vi "Force Anode Puge--SubVI.vi"(7 "Anode Request Events":T1, 8 "error in (no error)":errorcluster, 9 "Purge Settings in":T4, 10 "Purge State in":T3, 11 "Refnum in":refnum<k21>) -> (0 "error out":errorcluster, 1 "Purge Settings out":T4, 2 "Purge State out 2":T3, 3 "Refnum out":refnum<k21>)   [LabVIEW 2024, in "Anode.lvlib"]
uses:
  Anode.lvlib
  Purge Strategy--cluster.ctl
  Purge Strategy--enum.ctl
  Purge Valve State--cluster.ctl
  Request Events--cluster.ctl
  Stop Argument--cluster.ctl
  Show Panel Argument--cluster.ctl
  Hide Panel Argument--cluster.ctl
  Get Module Execution Status Argument--cluster.ctl
  Show Diagram Argument--cluster.ctl
  Change Panel Argument--cluster.ctl
  <vilib>/MGI/Panel Manager/Panel/Panel/Panel.lvclass
  Set Anode Inlet Pressure SP Argument--cluster.ctl
  Initialise Pressure Regulator Interface Argument--cluster.ctl
  Modbus Config--cluster.ctl
  Start Polling Pressure Regulator Status Argument--cluster.ctl
  Stop Polling Pressure Regulator Status Argument--cluster.ctl
  Read Pressure Regulator Status Argument--cluster.ctl
  Set Pressure Regulator Control Function Argument--cluster.ctl
  Modbus Flexi-Flow API/Control Function Values--enum.ctl
  Set Anode Inlet Flow SP Argument--cluster.ctl
  Set Anode Inlet Valve State Argument--cluster.ctl
  Anode Solenoid Valve--enum.ctl
  Wake Connection Helper Loop Argument--cluster.ctl
  Set Anode Gas Supply Valve Argument--cluster.ctl
  Set Purge Valve Argument--cluster.ctl
  Set Purge Strategy Argument--cluster.ctl
  Wake Purge Strategy Helper Loop Argument--cluster.ctl
  Update Purge Strategy Settings Argument--cluster.ctl
  Wake Purge Helper Loop Argument--cluster.ctl
  Wake Recirculation Pump Helper Loop Argument--cluster.ctl
  Sleep Recirculation Pump Helper Loop Argument--cluster.ctl
  Set Pump Speed SP Argument--cluster.ctl
  Set Pump Enable State Argument--cluster.ctl
  Set Pump Speed Control Mode Argument--cluster.ctl
  Update Purge Strategy Helper Loop Argument--cluster.ctl
  Force Purge Argument--cluster.ctl
  Reset Counter Argument--cluster.ctl
  Wake H2 Sensor Loop Argument--cluster.ctl
  Sleep H2 Sensor Loop Argument--cluster.ctl
  Start H2 Sensor Measurement Argument--cluster.ctl
  Stop H2 Sensor Measurement Argument--cluster.ctl
  <vilib>/DAQmx/write.llb/DAQmx Write (Digital Bool 1Line 1Point).vi
  <vilib>/DAQmx/miscellaneous.llb/DAQmx Fill In Error Info.vi
  Modbus Flexi-Flow API/Bronkhorst Flexi-Flow ModbusTCP API.lvlib
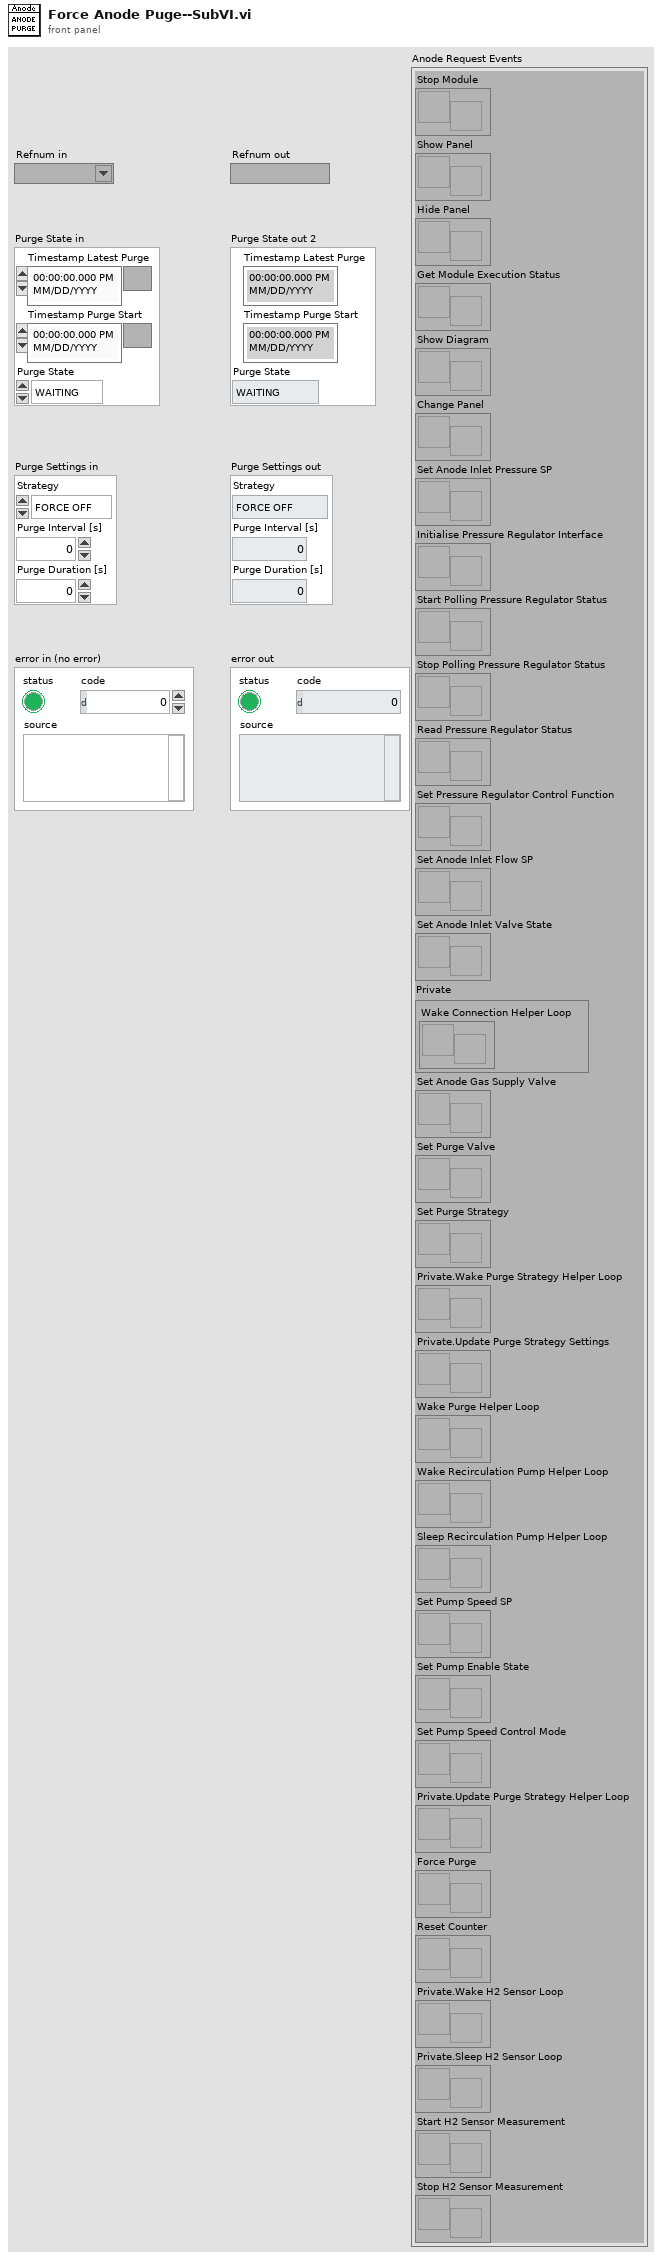
[diagram p1: front panel]
types:
  T1 = typedef "Anode.lvlib/Request Events--cluster.ctl" = cluster{"Stop Module":refnum<user-event>, "Show Panel":refnum<user-event>, "Hide Panel":refnum<user-event>, "Get Module Execution Status":refnum<user-event>, "Show Diagram":refnum<user-event>, "Change Panel":refnum<user-event>, "Set Anode Inlet Pressure SP":refnum<user-event>, "Initialise Pressure Regulator Interface":refnum<user-event>, "Start Polling Pressure Regulator Status":refnum<user-event>, "Stop Polling Pressure Regulator Status":refnum<user-event>, "Read Pressure Regulator Status":refnum<user-event>, "Set Pressure Regulator Control Function":refnum<user-event>, "Set Anode Inlet Flow SP":refnum<user-event>, "Set Anode Inlet Valve State":refnum<user-event>, "Private":cluster{"Wake Connection Helper Loop":refnum<user-event>}, "Set Anode Gas Supply Valve":refnum<user-event>, "Set Purge Valve":refnum<user-event>, "Set Purge Strategy":refnum<user-event>, "Private.Wake Purge Strategy Helper Loop":refnum<user-event>, "Private.Update Purge Strategy Settings":refnum<user-event>, "Wake Purge Helper Loop":refnum<user-event>, "Wake Recirculation Pump Helper Loop":refnum<user-event>, "Sleep Recirculation Pump Helper Loop":refnum<user-event>, "Set Pump Speed SP":refnum<user-event>, "Set Pump Enable State":refnum<user-event>, "Set Pump Speed Control Mode":refnum<user-event>, "Private.Update Purge Strategy Helper Loop":refnum<user-event>, "Force Purge":refnum<user-event>, "Reset Counter":refnum<user-event>, "Private.Wake H2 Sensor Loop":refnum<user-event>, "Private.Sleep H2 Sensor Loop":refnum<user-event>, "Start H2 Sensor Measurement":refnum<user-event>, "Stop H2 Sensor Measurement":refnum<user-event>}
  T2 = typedef "Anode.lvlib/Purge Valve State--cluster.ctl" = enum16{"WAITING", "PURGING"}
  T3 = cluster{"Timestamp Latest Purge":timestamp, "Timestamp Purge Start":timestamp, "Purge State":T2}
  T4 = typedef "Anode.lvlib/Purge Strategy--cluster.ctl" = cluster{"Strategy":T5, "Purge Interval [s]":dbl, "Purge Duration [s]":dbl}
  T5 = typedef "Anode.lvlib/Purge Strategy--enum.ctl" = enum16{"FORCE OFF", "FORCE ON", "TIMED"}
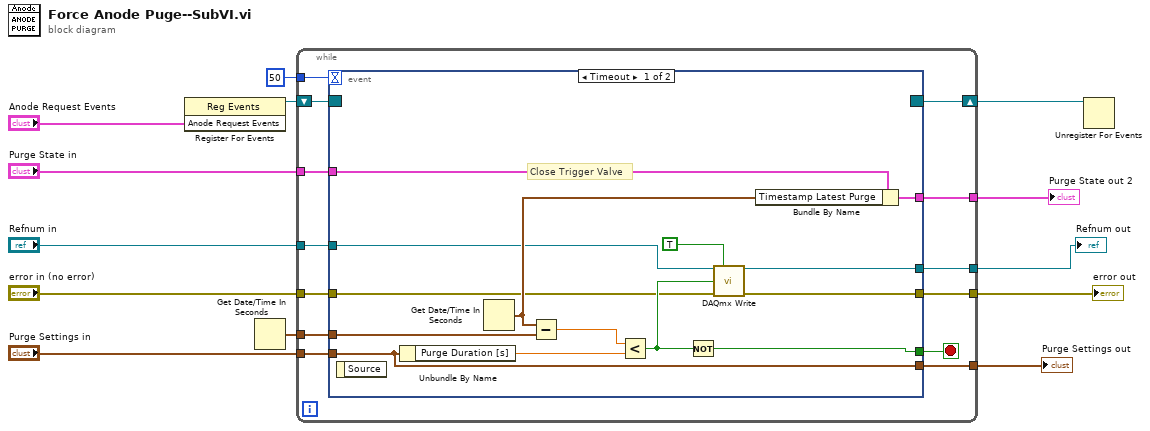
[diagram p0: block diagram]
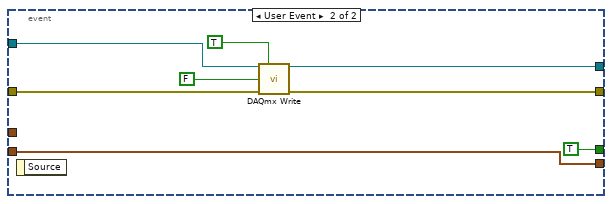
[diagram p2: hidden frame]
diagram:
  n1 = register-events ("DQMH_HELPER_REGFOREVENTS")("Anode Request Events") -> (reference out=w4:refnum<event-registration>)  [unwired: 2 in, 1 out]
  n2 = Get Date/Time In Seconds() -> (seconds since 1Jan1904=w2:timestamp)
  n3 = while {
    tunnel: [w26] -> w6
    tunnel: "Purge State in" -> [w25]
    tunnel: "Refnum in" -> [w21]
    tunnel: [w24] -> w9
    tunnel: "Purge Settings in" -> [w23]
    tunnel: [w19] -> w11
    tunnel: "error in (no error)" -> [w20]
    tunnel: [w22] -> w13
    tunnel: 50 -> [w17]
    tunnel: w2 -> [w16]
    shift-right: [w14] -> w1
    shift-left: w4 -> [w18]
    stop <- w15 stop-if-true
    n4 = event shown="[0] Timeout" {
      selector: w18 -> [_ _]
      dyn-events: [_ _] -> w14
      timeout: w17 -> [_ _]
      tunnel: [w34 _] -> w26
      tunnel: w25 -> [w35 _]
      tunnel: [w37 w41] -> w24
      tunnel: w23 -> [w37 w41]
      tunnel: [w27 w46] -> w22
      tunnel: w21 -> [w28 w45]
      tunnel: w20 -> [w30 w42]
      tunnel: [w29 w43] -> w19
      tunnel: w16 -> [w40 _]
      tunnel: [w31 TRUE ("auto start")] -> w15
      event Timeout {
        # "Close Trigger Valve"
        n5 = event-data() -> ()  [unwired: 1 in, 1 out]
        n6 = Unbundle By Name(w37) -> ("Purge Duration [s]"=w38:dbl)
        n7 = Get Date/Time In Seconds() -> (seconds since 1Jan1904=w33:timestamp)
        n8 = Subtract(x=w33, y=w40) -> (x-y=w36:dbl)
        n9 = Less?(x=w36, y=w38) -> (x < y?=w32:bool)
        n10 = Not(x=w32) -> (.not. x?=w31:bool)
        n11 = call-poly <vilib>:"DAQmx Write.vi"("task/channels in"=w28, "auto start"=TRUE, "data"=w32, "error in"=w30) -> ("task out"=w27:refnum<k21>, "error out"=w29:errorcluster)  [unwired: 9 in, 1 out]
        n12 = Bundle By Name(cluster=w35, "Timestamp Latest Purge"=w33) -> (w34:T3)
      }
      event User Event {
        n13 = event-data() -> ()  [unwired: 1 in, 1 out]
        n14 = call-poly <vilib>:"DAQmx Write.vi"("task/channels in"=w45, "auto start"=TRUE, "data"=FALSE, "error in"=w42) -> ("task out"=w46:refnum<k21>, "error out"=w43:errorcluster)  [unwired: 9 in, 1 out]
      }
    }
  }
  "Refnum out" <- w13
  "error out" <- w11
  "Purge Settings out" <- w9
  "Purge State out 2" <- w6
  n15 = Unregister For Events(event registration refnum=w1) -> ()  [unwired: 1 in, 1 out]
